vi "CheckCtlIsPresent.vi"(8 "error in (no error)":errorcluster, 11 "Message":T1) -> (0 "error out":errorcluster, 2 "ctl present":bool, 3 "Message":T1)   [LabVIEW 2017, in "MessageGen.lvlib"]
uses:
  <vilib>/addons/InsightCM/MessageBus/CodeGen/MessageGen.lvlib
  <vilib>/addons/InsightCM/MessageBus/CodeGen/controls/MessageData.ctl
  <vilib>/addons/InsightCM/MessageBus/CodeGen/controls/MessageType.ctl
  <vilib>/addons/InsightCM/MessageBus/CodeGen/controls/Parameter.ctl
  <vilib>/addons/InsightCM/MessageBus/CodeGen/controls/ParameterType.ctl
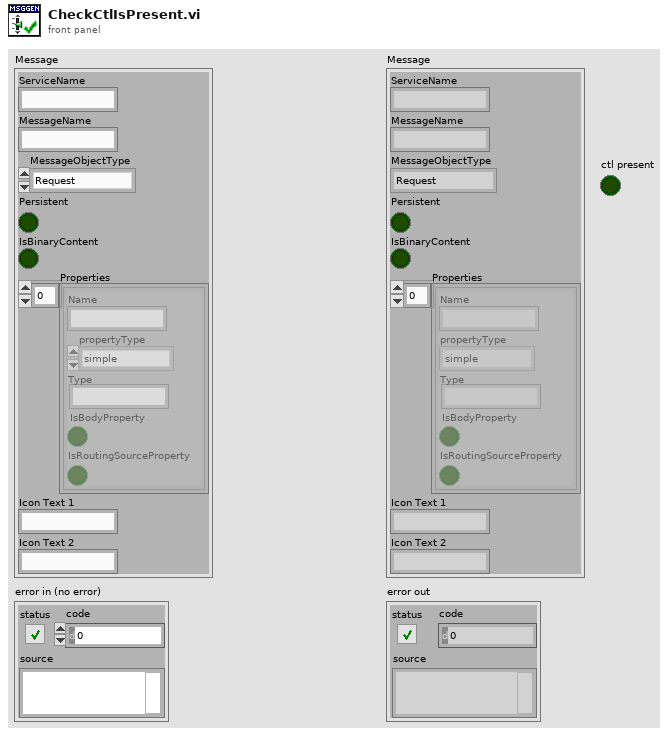
[diagram p1: front panel]
types:
  T1 = typedef "MessageGen.lvlib/MessageData.ctl" = cluster{"ServiceName":string, "MessageName":string, "MessageObjectType":T2, "Persistent":bool, "IsBinaryContent":bool, "Properties":T3[], "Icon Text 1":string, "Icon Text 2":string}
  T2 = typedef "MessageGen.lvlib/MessageType.ctl" = enum16{"Request", "Response", "Broadcast", "RoutedMessage"}
  T3 = typedef "MessageGen.lvlib/Parameter.ctl" = cluster{"Name":string, "propertyType":T4, "Type":string, "IsBodyProperty":bool, "IsRoutingSourceProperty":bool}
  T4 = typedef "MessageGen.lvlib/ParameterType.ctl" = enum16{"simple", "bytearray", "dateTime", "list", "map", "object"}
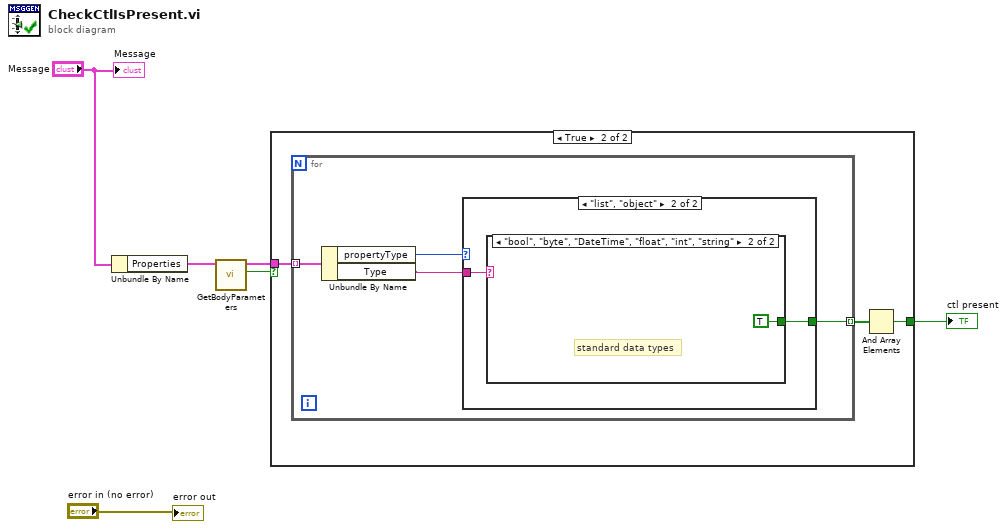
[diagram p0: block diagram]
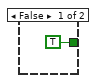
[diagram p2: hidden frame]
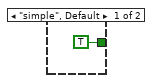
[diagram p3: hidden frame]
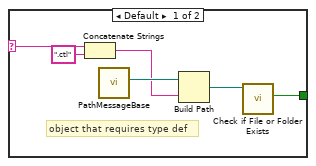
[diagram p4: hidden frame]
diagram:
  n1 = Unbundle By Name("Message") -> ("Properties"=w5:T3[])
  n2 = call <vilib>:"GetBodyParameters.vi"("Parameters"=w5) -> ("HasBodyParameters"=w2:bool, "BodyParameters"=w3:T3[])  [unwired: 9 in]
  n3 = case shown="True" w2 {
    tunnel: w3 -> [_ w10]
    tunnel: [TRUE w8] -> w1
    frame False {
    }
    frame True {
      n4 = for {
        tunnel: w10 -> [w12] mode=indexing
        tunnel: [w11] -> w9 mode=indexing
        n5 = Unbundle By Name(w12) -> ("propertyType"=w13:T4, "Type"=w14:string)
        n6 = case shown="\"list\", \"object\"" w13 {
          tunnel: w14 -> [_ w17]
          tunnel: [TRUE ("file or folder exists?") w16] -> w11
          frame "simple", Default {
          }
          frame "list", "object" {
            n7 = case shown="\"bool\", \"byte\", \"DateTime\", \"float\", \"int\", \"string\"" w17 {
              selector: w17 -> [w18 _]
              tunnel: [w19 TRUE ("file or folder exists?")] -> w16
              frame Default {
                # "object that requires type def"
                n8 = Concatenate Strings(w18, ".ctl" ("string")) -> (w21:string)
                n9 = call <vilib>:"PathMessageBase.vi"() -> ("Path"=w22:path)  [unwired: 11 in]
                n10 = Build Path(base path=w22, name or relative path=w21) -> (appended path=w23:path)
                n11 = call <vilib>:"Check if File or Folder Exists.vi"("path"=w23) -> ("file or folder exists?"=w19:bool)  [unwired: 8 in, 2 out]
              }
              frame "bool", "byte", "DateTime", "float", "int", "string" {
                # "standard data types"
              }
            }
          }
        }
      }
      n12 = And Array Elements(Boolean array=w9) -> (logical AND=w8:bool)
    }
  }
  "ctl present" <- w1
  "error out" <- "error in (no error)"
  "Message" <- "Message"
